vi "Draw.vi"(8 "error in (no error)":errorcluster, 11 "Square in":refnum<class "Square.lvclass">) -> (0 "error out":errorcluster, 2 "Shape":picture, 3 "Square out":refnum<class "Square.lvclass">)   [LabVIEW 2019, in "Square.lvclass"]
uses:
  Square.lvclass
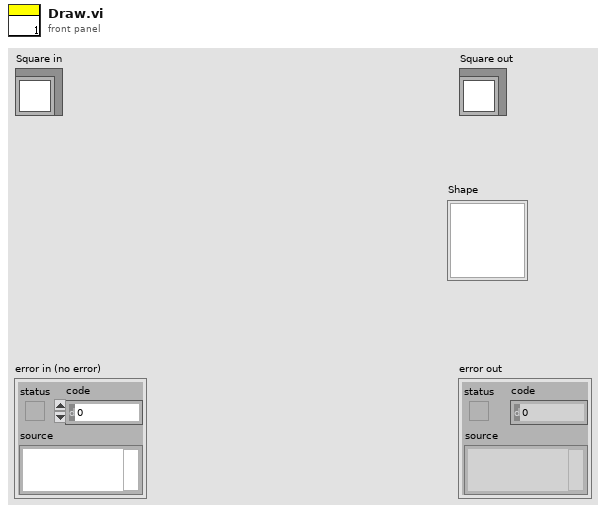
[diagram p1: front panel]
types:
  T1 = cluster{"left":i16, "top":i16, "right":i16, "bottom":i16}
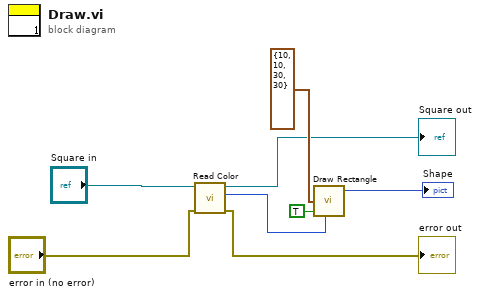
[diagram p0: block diagram]
diagram:
  n1 = call-dynamic "Read Color.vi"("error in (no error)"="error in (no error)", "Shape in"="Square in") -> ("error out"=→"error out":errorcluster, "Color"=w1:u32, "Shape out"=→"Square out":refnum<class "Square.lvclass">)  [unwired: 7 in]
  n2 = call <vilib>:"Draw Rectangle.vi"("rect"=T1 {"left"=10, "top"=10, "right"=30, "bottom"=30}, "fill?(F)"=TRUE, "color(black)"=w1) -> ("new picture"=→"Shape":picture)  [unwired: 6 in]
